vi "参考-读取制表符分隔的文件到显示为表格.vi"() -> ()   [LabVIEW 2018]
panel:
  out "数据表":string[][](table)
  out "数据图":dbl[][](graph)
  out "以制表符分隔的原始数据":string
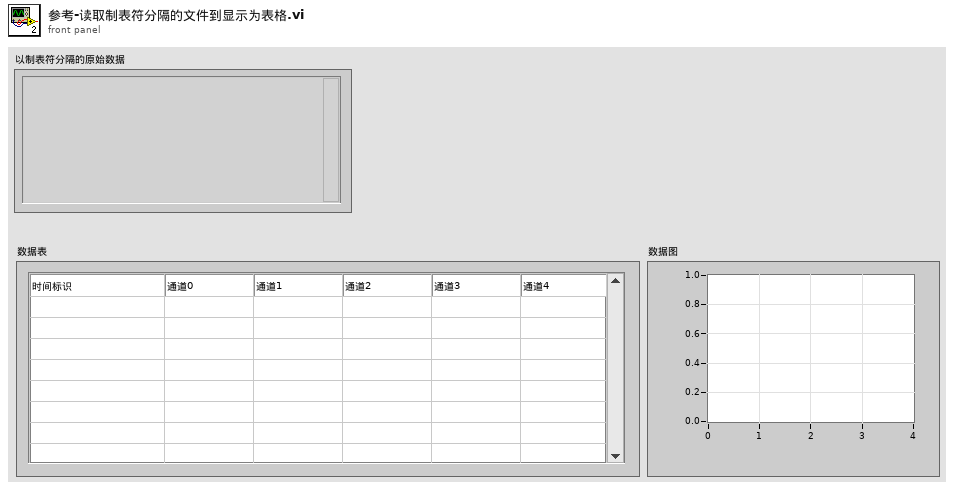
[diagram p1: front panel]
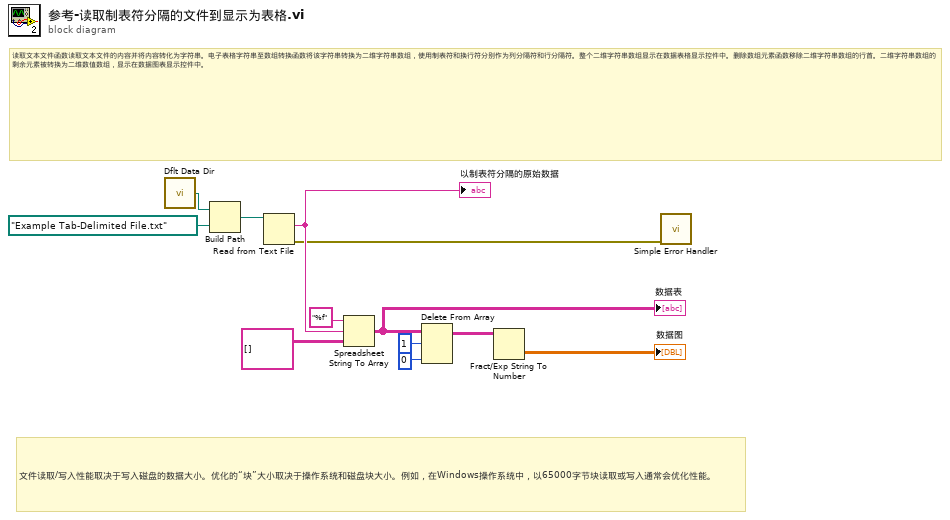
[diagram p0: block diagram]
diagram:
  # "文件读取/写入性能取决于写入磁盘的数据大小。优化的“块”大小取决于操作系统和磁盘块大小。例如，在Windows操作系统中，以65000字节块读取或写入通常会优化性能。"
  # "读取文本文件函数读取文本文件的内容并将内容转化为字符串。电子表格字符串至数组转换函数将该字符串转换为二维字符串数组，使用制表符和换行符分别作为列分隔符和行分隔符。整个二维字符串数组显示在数据表格显示控件中。删除数组元素函数移除二维字符串数组的行首。二维字符串数组的剩余元素被转换为二维数值数组，显示在数据图表显示控件中。"
  n1 = call <vilib>:"Dflt Data Dir.vi"() -> ("App:Default Data Directory"=w7:path)
  n2 = Build Path(base path=w7, name or relative path=path "Example Tab-Delimited File.txt" ("default name")) -> (appended path=w4:path)
  n3 = Read from Text File(file (use dialog)=w4) -> (text=w8:string, error out=w5:errorcluster)  [unwired: 2 in, 3 out]
  "以制表符分隔的原始数据" <- w8
  n4 = Spreadsheet String To Array(format string="%f", spreadsheet string=w8, array type (2D Dbl)=string[][] [] ("Array")) -> (array=w1:string[][])  [unwired: 1 in]
  "数据表" <- w1
  n5 = Delete From Array(array=w1, length=1, index (col)=0 ("disabled index (col)")) -> (array with subset deleted=w2:string[][])  [unwired: 1 in, 1 out]
  n6 = Fract/Exp String To Number(string=w2) -> (number=→"数据图":dbl[][])  [unwired: 4 out]
  n7 = call <vilib>:"Simple Error Handler.vi"("error in (no error)"=w5) -> ()  [unwired: 1 in, 8 out]
